vi "lvEtherbone.device_open.vi"(0 "eb_socket_ID":i32, 1 "address":string, 5 "error in (no error)":errorcluster) -> (13 "eb_status":T1 items=["EB_SUCCESS"=1, "EB_OK"=0, "EB_FAIL"=-1, "EB_ADDRESS"=-2, "EB_WIDTH"=-3, "EB_OVERFLOW"=-4, "EB_ENDIAN"=-5, "EB_BUSY"=-6, "EB_TIMEOUT"=-7, "EB_OOM"=-8, "EB_ABI"=-9, "EB_SEGFAULT"=-10], 14 "eb_socket_ID out":i32, 15 "eb_device_ID":i32, 19 "error out":errorcluster)   [LabVIEW 2012, in "lvEtherbone.lvlib"]
doc: "/* Open a remote Etherbone device at 'address' (default port 0xEBD0).\n * Negotiation of bus widths is attempted every 3 seconds, 'attempts' times.\n * The proposed_widths is intersected with the remote and local socket widths.\n * From the remaining widths, the largest address and data width is chosen.\n *\n * Return codes:\n * OK - the remote etherbone device is ready\n * ADDRESS - the network address could not be parsed\n * TIMEOUT - timeout waiting for etherbone response\n * FAIL - failure of the transport layer (remote host down?)\n * WIDTH - could not negotiate an acceptable data bus width\n * OOM - out of memory\n */\nEB_PUBLIC\neb_status_t eb_device_open(eb_socket_t socket,\n const char* address,\n eb_width_t proposed_widths,\n int attempts,\n eb_device_t* result);"
uses:
  lvEtherbone.lvlib
  lvEtherbone.lveb_status_t.ctl
  libetherbone.so
panel:
  in  "eb_status_t":T1 items=["EB_SUCCESS"=1, "EB_OK"=0, "EB_FAIL"=-1, "EB_ADDRESS"=-2, "EB_WIDTH"=-3, "EB_OVERFLOW"=-4, "EB_ENDIAN"=-5, "EB_BUSY"=-6, "EB_TIMEOUT"=-7, "EB_OOM"=-8, "EB_ABI"=-9, "EB_SEGFAULT"=-10]
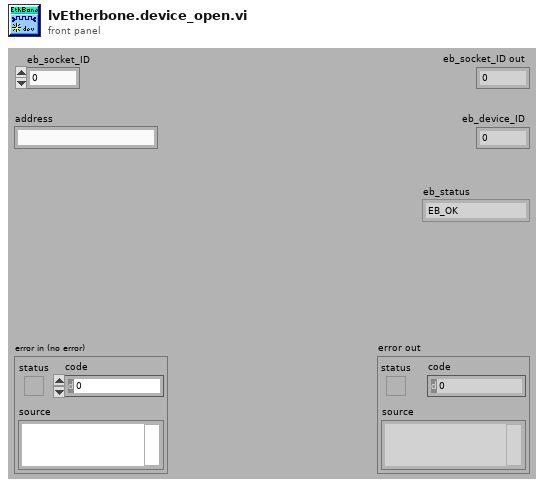
[diagram p1: front panel]
types:
  T1 = typedef "lvEtherbone.lvlib/lvEtherbone.lveb_status_t.ctl" = i32
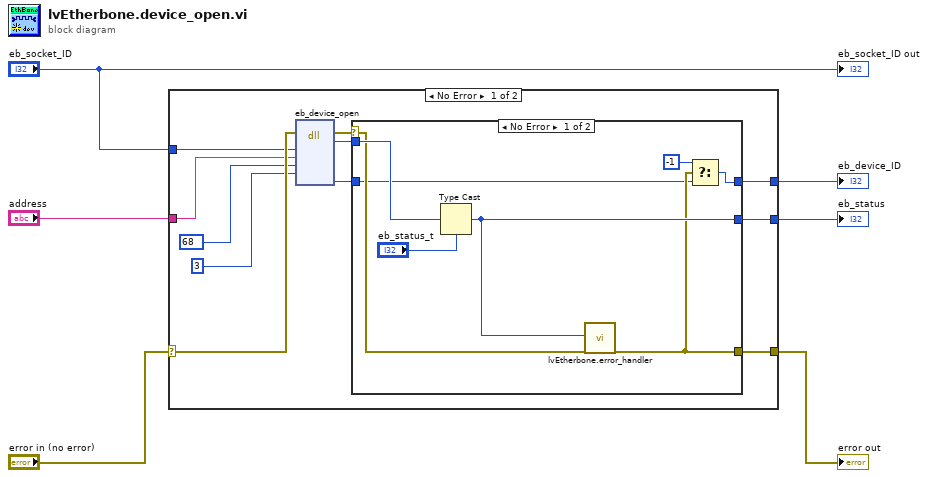
[diagram p0: block diagram]
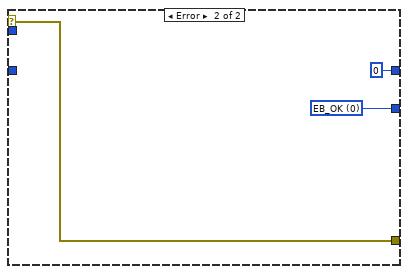
[diagram p2: hidden frame]
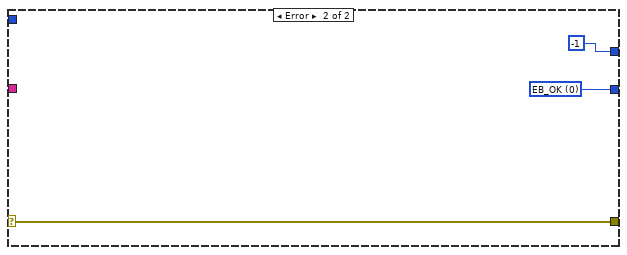
[diagram p3: hidden frame]
diagram:
  n1 = case shown="No Error" "error in (no error)" {
    selector: "error in (no error)" -> [w17 w31]
    tunnel: [w14 w31] -> w5
    tunnel: "eb_socket_ID" -> [w9 _]
    tunnel: "address" -> [w11 _]
    tunnel: [w15 w30] -> w3
    tunnel: [w13 -1 ("eb_socket_ID")] -> w2
    frame No Error {
      n2 = dll-call lib="libetherbone.so" fn="eb_device_open"(error in=w17, "eb_socket_ID"=w9, "address"=w11, "proposed_widths"=u8 68, "attempts"=3) -> (error out=w12:errorcluster, "eb_status"=w16:i32, "eb_device_ID"=w10:u16)  [unwired: 7 in, 1 out]
      n3 = case shown="No Error" w12 {
        selector: w12 -> [w23 w28]
        tunnel: w16 -> [w25 _]
        tunnel: [w22 w27] -> w15
        tunnel: [w19 w28] -> w14
        tunnel: w10 -> [w18 _]
        tunnel: [w21 u16 0 ("eb_device_ID")] -> w13
        frame No Error {
          n4 = Type Cast(type="eb_status_t", x=w25) -> (*(type *) &x=w22:T1)
          n5 = call "lvEtherbone.error_handler.vi"("eb_status"=w22, "error in"=w23) -> ("error out"=w19:errorcluster)  [unwired: 17 in]
          n6 = Select(t=-1 ("eb_device_ID"), s=w19, f=w18) -> (s? t:f=w21:i32)
        }
        frame Error {
          w27 = T1 0 items=["EB_SUCCESS"=1, "EB_OK"=0, "EB_FAIL"=-1, "EB_ADDRESS"=-2, "EB_WIDTH"=-3, "EB_OVERFLOW"=-4, "EB_ENDIAN"=-5, "EB_BUSY"=-6, "EB_TIMEOUT"=-7, "EB_OOM"=-8, "EB_ABI"=-9, "EB_SEGFAULT"=-10] ("eb_status_t")
        }
      }
    }
    frame Error {
      w30 = T1 0 items=["EB_SUCCESS"=1, "EB_OK"=0, "EB_FAIL"=-1, "EB_ADDRESS"=-2, "EB_WIDTH"=-3, "EB_OVERFLOW"=-4, "EB_ENDIAN"=-5, "EB_BUSY"=-6, "EB_TIMEOUT"=-7, "EB_OOM"=-8, "EB_ABI"=-9, "EB_SEGFAULT"=-10] ("eb_status_t")
    }
  }
  "error out" <- w5
  "eb_status" <- w3
  "eb_device_ID" <- w2
  "eb_socket_ID out" <- "eb_socket_ID"
